vi "Close.vi"(8 "error in (no error)":errorcluster, 11 "CellStyle in":refnum<class "CellStyle.lvclass">) -> (0 "error out":errorcluster)   [LabVIEW 2013, in "DataGrid.lvlib" / "CellStyle.lvclass"]
uses:
  CellStyle.lvclass
  CellStyle.lvclass/CellStyle.ctl
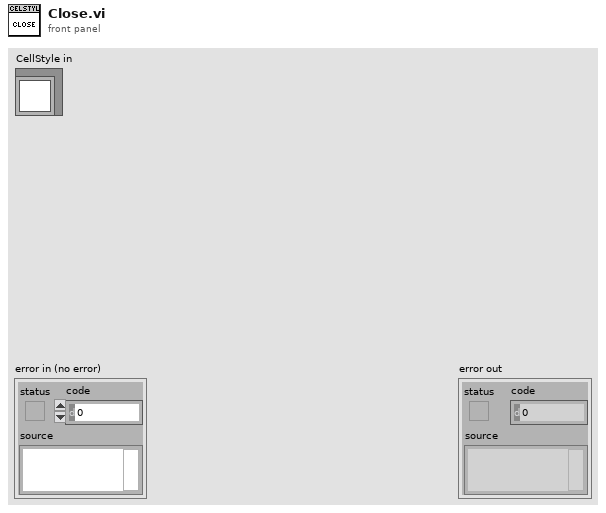
[diagram p1: front panel]
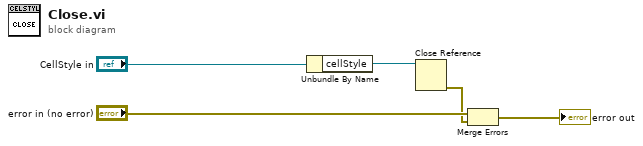
[diagram p0: block diagram]
diagram:
  n1 = Unbundle By Name("CellStyle in") -> ("cellStyle"=w1:refnum<k24>)
  n2 = Close Reference(reference=w1) -> (error out=w3:errorcluster)  [unwired: 1 in]
  n3 = Merge Errors("error in (no error)", w3) -> (→"error out":errorcluster)
